vi "Result All Steps Judgement Codes.vi"(8 "error in (no error)":errorcluster, 11 "VISA resource name":refnum<visa-resource-name>) -> (0 "error out":errorcluster, 2 "Results":string, 3 "VISA resource name out":refnum<visa-resource-name>)   [LabVIEW 2025, in "Chroma 19572.lvlib"]
uses:
  <instrlib>/Chroma 19572/Chroma 19572.lvlib
panel:
  # "All Steps Judgement Codes Results query"
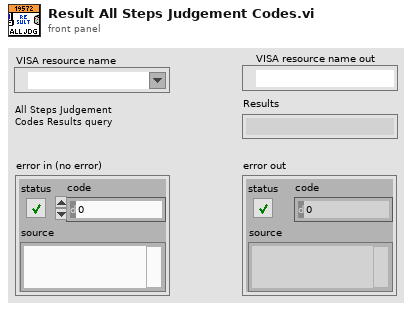
[diagram p1: front panel]
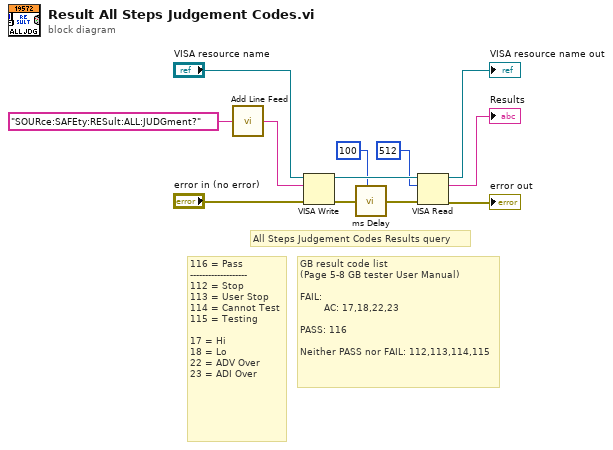
[diagram p0: block diagram]
diagram:
  # "GB result code list \n(Page 5-8 GB tester User Manual)\n\nFAIL: \n        AC: 17,18,22,23\n\nPASS: 116\n\nNeither PASS nor FAIL: 112,113,114,115"
  # "116 = Pass\n-------------------\n112 = Stop\n113 = User Stop\n114 = Cannot Test\n115 = Testing\n\n17 = Hi\n18 = Lo\n22 = ADV Over\n23 = ADI Over"
  # "All Steps Judgement Codes Results query"
  n1 = call <instrlib>:"Add Line Feed.vi"("Command string"="SOURce:SAFEty:RESult:ALL:JUDGment?") -> ("Concatenated string"=w1:string)  [unwired: 4 in]
  n2 = VISA Write(VISA resource name="VISA resource name", write buffer=w1, error in (no error)="error in (no error)") -> (VISA resource name out=w12:refnum<visa-resource-name>, error out=w7:errorcluster)  [unwired: 1 out]
  n3 = call <instrlib>:"ms Delay.vi"("miliseconds to wait"=u32 100, "error in (no error)"=w7) -> ("error out"=w6:errorcluster)  [unwired: 6 in, 1 out]
  n4 = VISA Read(VISA resource name=w12, byte count=u32 512, error in (no error)=w6) -> (VISA resource name out=→"VISA resource name out":refnum<visa-resource-name>, read buffer=→"Results":string, error out=→"error out":errorcluster)  [unwired: 1 out]
